vi "MenuExamples.vi"() -> ()   [LabVIEW 2023]
panel:
  in  "stop":bool
  in  "vi path":path
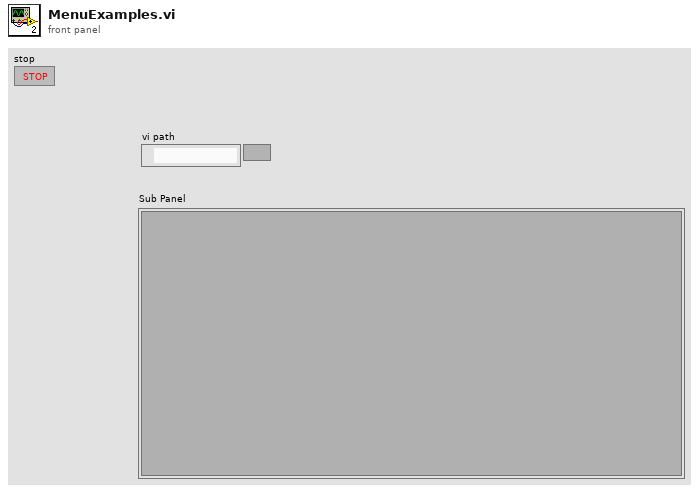
[diagram p1: front panel]
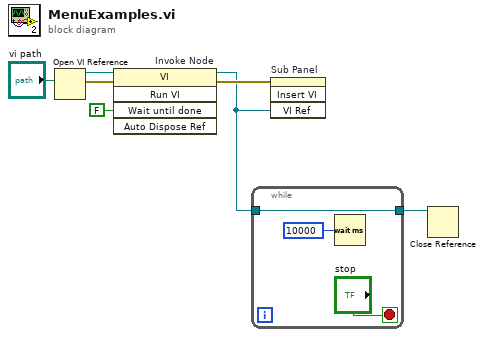
[diagram p0: block diagram]
diagram:
  n1 = Open VI Reference(vi path="vi path") -> (vi reference=w6:refnum<vi>, error out=w4:errorcluster)  [unwired: 5 in]
  n2 = invoke on="Invoke Node" class="VI" method="Run VI"(reference=w6, error in=w4, "Wait until done"=FALSE ("Wait Until Done")) -> (reference out=w2:refnum<vi>, error out=w5:errorcluster)  [unwired: 2 in, 3 out]
  n3 = while {
    tunnel: w2 -> [w8]
    tunnel: [w8] -> w1
    stop <- "stop" stop-if-true
    n4 = Wait (ms)(milliseconds to wait=u32 10000) -> ()  [unwired: 1 out]
  }
  n5 = invoke on="Sub Panel" class="SubPnl" method="Insert VI"(error in=w5, "VI Ref"=w2) -> ()  [unwired: 2 in, 4 out]
  n6 = Close Reference(reference=w1) -> ()  [unwired: 1 in, 1 out]
